vi "Test Error Propagation.vi"(11 "Test Case In":refnum<class "Test Open Xml.lvclass">) -> (0 "error out":errorcluster, 3 "Test Case Out":refnum<class "Test Open Xml.lvclass">)   [LabVIEW 2020, in "Test Open Xml.lvclass"]
uses:
  Test Open Xml.lvclass
  Source/Open Xml.lvlib
  5b340422-defb-4753-92ae-10f5ae7bb3d8.vi
  de3616c6-4837-4eef-92cf-f4a5127a2287.vi
  f757fa54-b07b-4a92-a289-7ce739c836a6.vi
  <vilib>/numeric/Random Number (Range) DBL.vi
  0ce37261-f17c-4487-8556-4dec27feb262.vi
  dbe47212-de57-4456-ba1d-2209d4b44483.vi
  4b527410-3829-466b-86c3-b8d1fd0707f5.vi
  a2e1416a-ebe4-4e53-9655-ad8087ccd270.vi
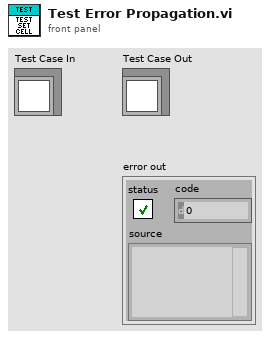
[diagram p1: front panel]
types:
  T1 = enum16{"Boolean", "Number", "Error", "SharedString", "String", "InlineString", "Date"}
  T2 = enum16{"Boolean", "Number", "Error", "SharedString", "String", "InlineString", "Date"}[]
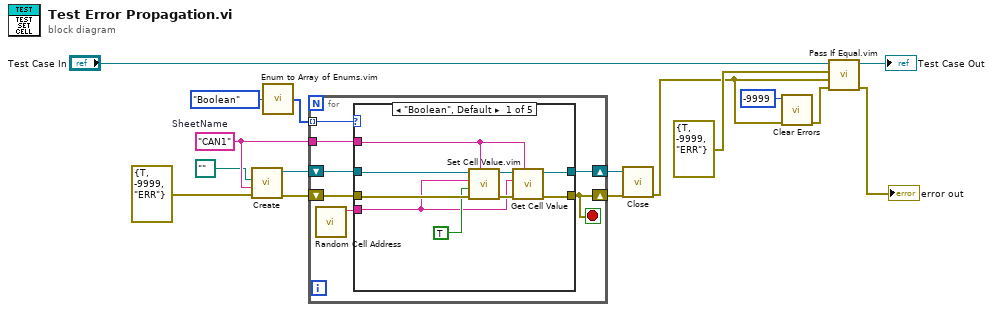
[diagram p0: block diagram]
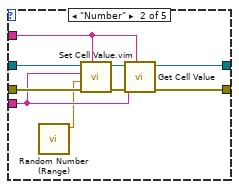
[diagram p2: hidden frame]
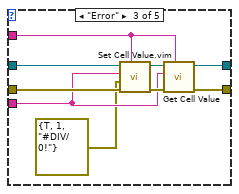
[diagram p3: hidden frame]
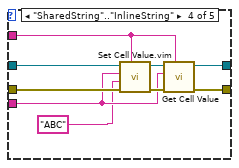
[diagram p4: hidden frame]
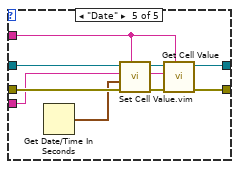
[diagram p5: hidden frame]
diagram:
  w9 = "CAN1"  # SheetName
  n1 = call "Create.vi"("error in"=errorcluster {"status"=TRUE, "code"=-9999, "source"="ERR"}, "SheetName"=w9, "Path"=path "") -> ("error out"=w12:errorcluster, "SpreadsheetDoc"=w13:refnum<k24>)  [unwired: 7 in]
  n2 = call "Enum to Array of Enums.vim"("enum"=T1."Boolean") -> ("array of enums"=w7:T2)
  n3 = for {
    tunnel: w9 -> [w20]
    shift-right: [w21] -> w10
    shift-left: w13 -> [w23]
    shift-right: [w18] -> w11
    shift-left: w12 -> [w22]
    tunnel: w7 -> [w19] mode=indexing
    stop <- w18 stop-if-true
    n4 = call "Random Cell Address.vi"() -> ("Random Cell Address"=w17:string)  [unwired: 11 in]
    n5 = case shown="\"Boolean\", Default" w19 {
      tunnel: w23 -> [w29 w41 w50 w59 w68]
      tunnel: w22 -> [w28 w40 w49 w58 w67]
      tunnel: [w26 w38 w47 w56 w65] -> w18
      tunnel: [w25 w36 w45 w54 w63] -> w21
      tunnel: w20 -> [w30 w35 w44 w53 w62]
      tunnel: w17 -> [w24 w34 w43 w52 w61]
      frame "Boolean", Default {
        n6 = call "Set Cell Value.vim"("Sheet Name"=w30, "error in"=w28, "Value"=TRUE, "Cell Address"=w24, "SpreadsheetDoc in"=w29) -> ("error out"=w32:errorcluster, "SpreadsheetDoc out"=w31:refnum<k24>)  [unwired: 5 in]
        n7 = call "Get Cell Value.vi"("Sheet Name"=w30, "error in"=w32, "Cell Address"=w24, "SpreadsheetDoc in"=w31) -> ("error out"=w26:errorcluster, "SpreadsheetDoc out"=w25:refnum<k24>)  [unwired: 4 in, 2 out]
      }
      frame "Number" {
        n8 = call-poly <vilib>:"Random Number (Range).vi"() -> ("number"=w33:dbl)  [unwired: 11 in]
        n9 = call "Set Cell Value.vim"("Sheet Name"=w35, "error in"=w40, "Value"=w33, "Cell Address"=w34, "SpreadsheetDoc in"=w41) -> ("error out"=w39:errorcluster, "SpreadsheetDoc out"=w37:refnum<k24>)  [unwired: 5 in]
        n10 = call "Get Cell Value.vi"("Sheet Name"=w35, "error in"=w39, "Cell Address"=w34, "SpreadsheetDoc in"=w37) -> ("error out"=w38:errorcluster, "SpreadsheetDoc out"=w36:refnum<k24>)  [unwired: 4 in, 2 out]
      }
      frame "Error" {
        n11 = call "Set Cell Value.vim"("Sheet Name"=w44, "error in"=w49, "Value"=errorcluster {"status"=TRUE, "code"=1, "source"="#DIV/0!"} ("error constant"), "Cell Address"=w43, "SpreadsheetDoc in"=w50) -> ("error out"=w48:errorcluster, "SpreadsheetDoc out"=w46:refnum<k24>)  [unwired: 5 in]
        n12 = call "Get Cell Value.vi"("Sheet Name"=w44, "error in"=w48, "Cell Address"=w43, "SpreadsheetDoc in"=w46) -> ("error out"=w47:errorcluster, "SpreadsheetDoc out"=w45:refnum<k24>)  [unwired: 4 in, 2 out]
      }
      frame "SharedString".."InlineString" {
        n13 = call "Set Cell Value.vim"("Sheet Name"=w53, "error in"=w58, "Value"="ABC", "Cell Address"=w52, "SpreadsheetDoc in"=w59) -> ("error out"=w57:errorcluster, "SpreadsheetDoc out"=w55:refnum<k24>)  [unwired: 5 in]
        n14 = call "Get Cell Value.vi"("Sheet Name"=w53, "error in"=w57, "Cell Address"=w52, "SpreadsheetDoc in"=w55) -> ("error out"=w56:errorcluster, "SpreadsheetDoc out"=w54:refnum<k24>)  [unwired: 4 in, 2 out]
      }
      frame "Date" {
        n15 = Get Date/Time In Seconds() -> (seconds since 1Jan1904=w60:timestamp)
        n16 = call "Set Cell Value.vim"("Sheet Name"=w62, "error in"=w67, "Value"=w60, "Cell Address"=w61, "SpreadsheetDoc in"=w68) -> ("error out"=w66:errorcluster, "SpreadsheetDoc out"=w64:refnum<k24>)  [unwired: 5 in]
        n17 = call "Get Cell Value.vi"("Sheet Name"=w62, "error in"=w66, "Cell Address"=w61, "SpreadsheetDoc in"=w64) -> ("error out"=w65:errorcluster, "SpreadsheetDoc out"=w63:refnum<k24>)  [unwired: 4 in, 2 out]
      }
    }
  }
  n18 = call "Close.vi"("error in"=w11, "SpreadsheetDoc"=w10) -> ("error out"=w3:errorcluster)  [unwired: 9 in]
  n19 = call <vilib>:"Clear Errors.vi"("error in (no error)"=w3, "specific error code to clear (0: all)"=-9999) -> ("error out"=w2:errorcluster)  [unwired: 4 in, 1 out]
  n20 = call "Pass If Equal.vim"("error in (no error)"=w2, "Actual"=w3, "Expected"=errorcluster {"status"=TRUE, "code"=-9999, "source"="ERR"} ("error constant"), "LUnit Test Case In"="Test Case In") -> ("error out"=→"error out":errorcluster, "LUnit Test Case Out"=→"Test Case Out":refnum<class "Test Open Xml.lvclass">)  [unwired: 6 in]
